vi "Autonomous Independent.vi"() -> ()   [LabVIEW 2015]
doc: "This VI is called when autonomous begins, and will automatically be terminated when autonomous ends. You can carry out timed or sensor driven robot movement independently without needing to return to the caller."
uses:
  <vilib>/Rock Robotics/WPI/Utilities/WPI_GetSetVariantRefNum.vi
  <vilib>/Rock Robotics/Network Tables/NT Write Numeric Array.vi
  <vilib>/Rock Robotics/Network Tables/NT Read String.vi
  <vilib>/Rock Robotics/WPI/RobotDrive/WPI_RobotDriveArcadeDrive_Standard(NoSaturation).vi
panel:
  out "Current Movement, for debugging":T1 {"Y Joystick Value" scale=1.0..-1.0; "X Joystick Value" scale=-1.0..1.0}
  in  "Array of robot movements":T2(array[cluster])=[{"X Joystick Value"=0.39393939393939403, "Y Joystick Value"=0.0, "Delay (sec)"=1.0, "Movement Name"="turn"}, {"X Joystick Value"=-0.3737373737373737, "Y Joystick Value"=0.0, "Delay (sec)"=1.0, "Movement Name"="turn back"}] {"Y Joystick Value" scale=1.0..-1.0; "X Joystick Value" scale=-1.0..1.0}
  # "Be sure to right-click and choose Data Operations>>Make Current Value default if you want to save the array values with the VI"
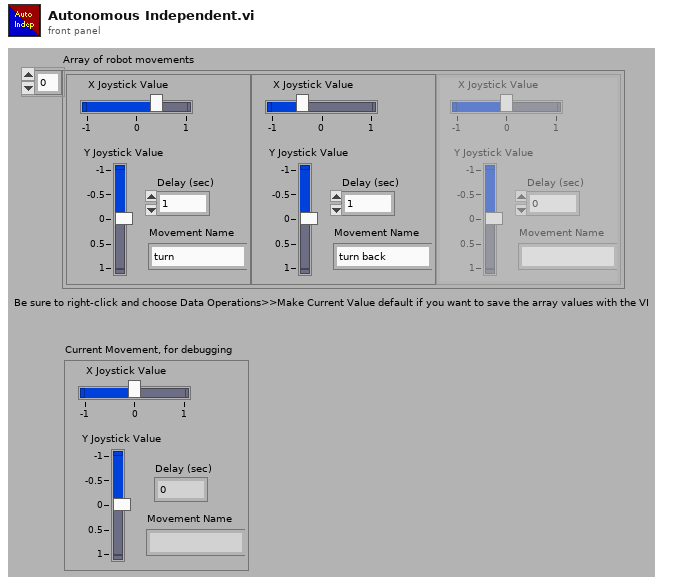
[diagram p1: front panel]
types:
  T1 = cluster{"X Joystick Value":dbl, "Y Joystick Value":dbl, "Delay (sec)":dbl, "Movement Name":string}
  T2 = cluster{"X Joystick Value":dbl, "Y Joystick Value":dbl, "Delay (sec)":dbl, "Movement Name":string}[]
  T3 = typedef "WPI_JoystickDevRef.ctl" = cluster{"Device":T4}
  T4 = typedef "WPI_JoystickDeviceEnum.ctl" = enum16{"USB 0", "USB 1", "USB 2", "USB 3", "USB 4", "USB 5"}
  T5 = typedef "WPI_RobotDriveDevRef.ctl" = cluster{"DevStatus":errorcluster, "Motors[]":T6[], "Square Inputs":bool, "Max Output":dbl}
  T6 = typedef "WPI_MotorControlDeviceRef.ctl" = cluster{"DeviceStatus":errorcluster, "Type":T7, "PWM":cluster{"PWM Channel":T8, "DeadBand":T9}, "CAN":cluster{"Device Number":u8, "Control Mode":T10, "Semaphore":T11, "Max Vout":dbl, "TalonSRX Control Mode":T12}, "Invert":bool}
  T7 = typedef "WPI_MotorControlType.ctl" = enum16{"PWM", "CAN", "CANTalonSRX"}
  T8 = typedef "FPGA_DIOPWMChannel.ctl" = enum8{"PWM 0", "PWM 1", "PWM 2", "PWM 3", "PWM 4", "PWM 5", "PWM 6", "PWM 7", "PWM 8", "PWM 9", "PWM MXP 0", "PWM MXP 1", "PWM MXP 2", "PWM MXP 3", "PWM MXP 4", "PWM MXP 5", "PWM MXP 6", "PWM MXP 7", "PWM MXP 8", "PWM MXP 9", "Invalid"}
  T9 = typedef "WPI_PWMDeadband.ctl" = cluster{"Name":string, "maxPositivePwm":i32, "minPositivePwm":i32, "centerPwm":i32, "maxNegativePwm":i32, "minNegativePwm":i32, "angularRange":u16}
  T10 = typedef "WPI_CANJaguar_ControlMode.ctl" = enum8{"Percent VBus", "Current", "Speed", "Position", "Voltage"}
  T11 = typedef "Semaphore RefNum" = refnum<k1>
  T12 = typedef "WPI_CANTalonSRX_APIControlMode.ctl" = enum8{"Percent VBus", "Speed", "Position", "Slave", "Unchanged / Invalid", "Voltage Compensation", "Current", "Motion Profile"}
  T13 = typedef "WPI_PotentiometerDevRef.ctl" = cluster{"DevStatus":errorcluster, "Analog Channel":T14, "Invert Output":bool}
  T14 = typedef "FPGA_AIChannel.ctl" = enum8{"AI 0", "AI 1", "AI 2", "AI 3", "AI MXP 0", "AI MXP 1", "AI MXP 2", "AI MXP 3", "Invalid"}
  T15 = typedef "WPI_SwitchDevRef.ctl" = cluster{"DevStatus":errorcluster, "DIO Channel":T16, "CntIndex":T17, "Normally Closed":bool}
  T16 = typedef "FPGA_DIOChannel.ctl" = enum8{"DIO 0", "DIO 1", "DIO 2", "DIO 3", "DIO 4", "DIO 5", "DIO 6", "DIO 7", "DIO 8", "DIO 9", "DIO MXP 0", "DIO MXP 1", "DIO MXP 2", "DIO MXP 3", "DIO MXP 4", "DIO MXP 5", "DIO MXP 6", "DIO MXP 7", "DIO MXP 8", "DIO MXP 9", "DIO MXP 10", "DIO MXP 11", "DIO MXP 12", "DIO MXP 13", "DIO MXP 14", "DIO MXP 15", "Invalid"}
  T17 = typedef "FPGA_CounterCtrSystemIndex.ctl" = enum8{"Ctr 0", "Ctr 1", "Ctr 2", "Ctr 3", "Ctr 4", "Ctr 5", "Ctr 6", "Ctr 7", "Invalid"}
  T18 = typedef "WPI_SolenoidDevRef.ctl" = cluster{"DevStatus":errorcluster, "Pneumatics Control Module":u8, "Forward Solenoid Channel":T19, "Reverse Solenoid Channel":T19}
  T19 = typedef "WPI_SolenoidChannel.ctl" = enum8{"Solenoid 0", "Solenoid 1", "Solenoid 2", "Solenoid 3", "Solenoid 4", "Solenoid 5", "Solenoid 6", "Solenoid 7", "Invalid"}
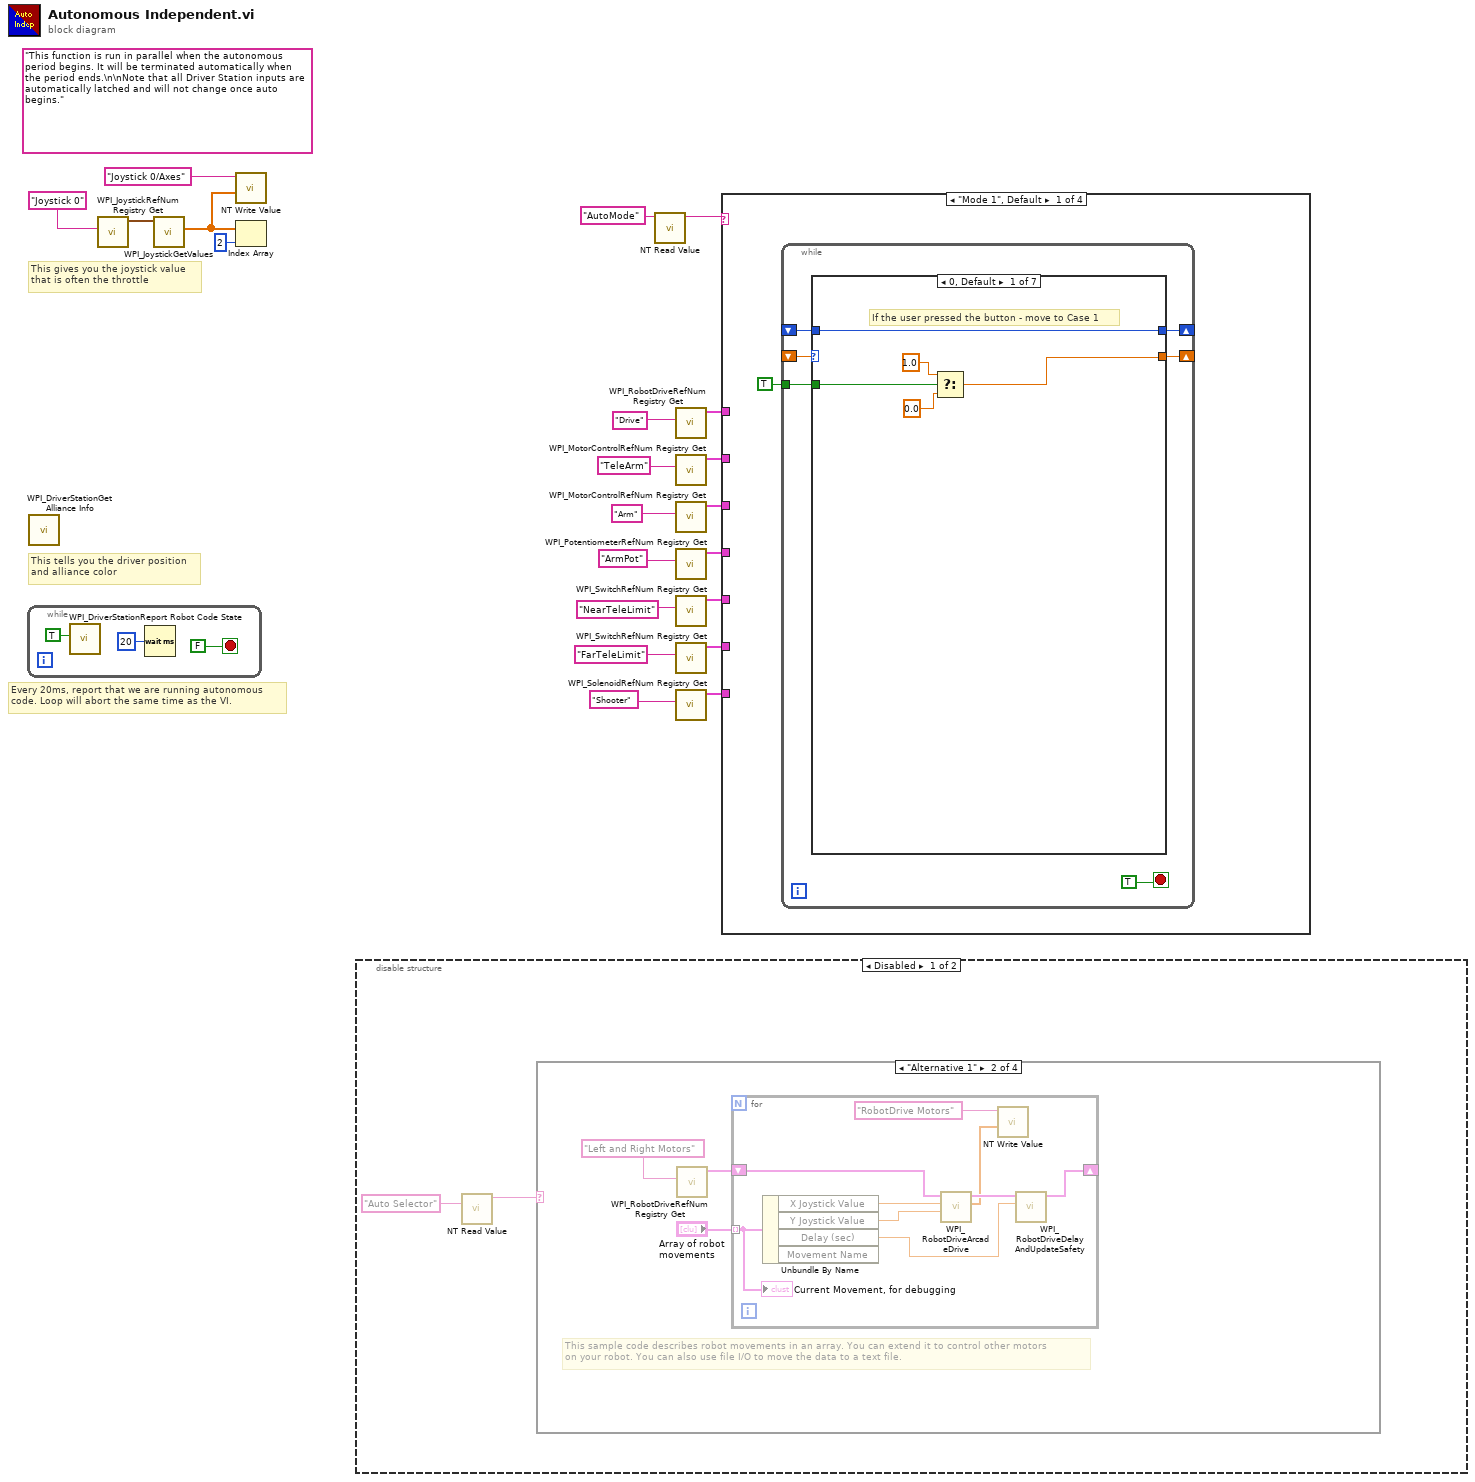
[diagram p0: block diagram]
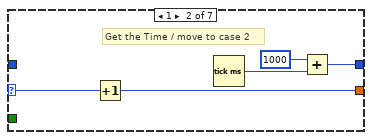
[diagram p2: hidden frame]
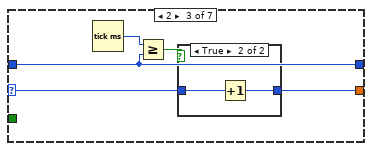
[diagram p3: hidden frame]
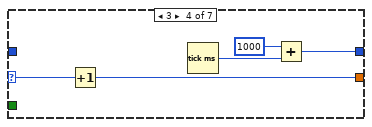
[diagram p5: hidden frame]
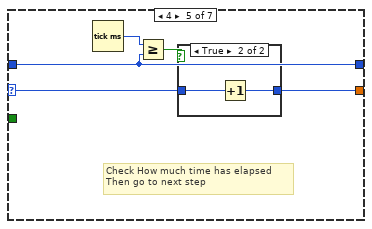
[diagram p6: hidden frame]
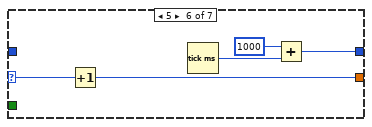
[diagram p8: hidden frame]
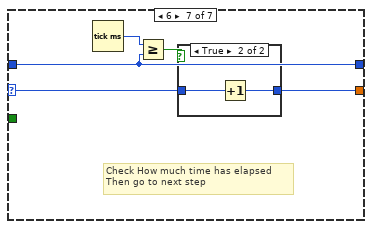
[diagram p9: hidden frame]
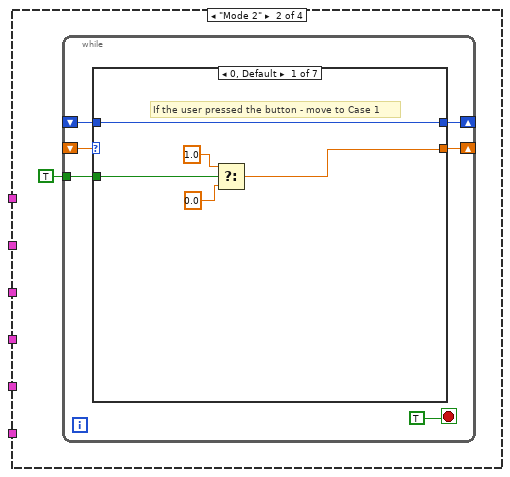
[diagram p11: hidden frame]
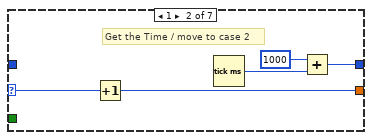
[diagram p12: hidden frame]
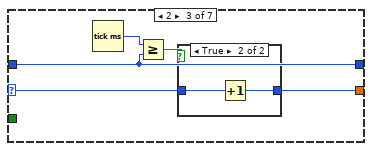
[diagram p13: hidden frame]
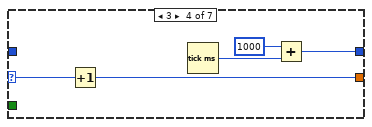
[diagram p15: hidden frame]
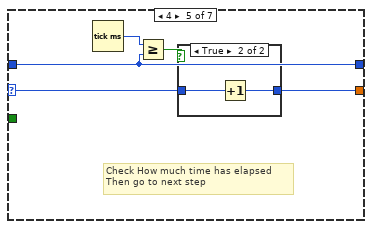
[diagram p16: hidden frame]
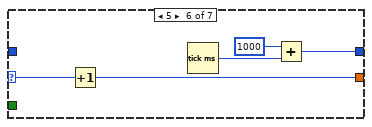
[diagram p18: hidden frame]
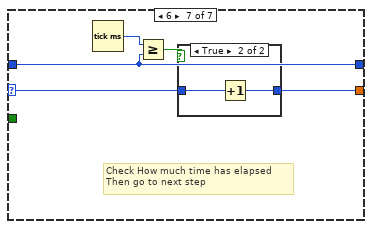
[diagram p19: hidden frame]
diagram:
  (unwired) "This function is run in parallel when the autonomous period begins. It will be terminated automatically when the period ends.\n\nNote that all Driver Station inputs are automatically latched and will not change once auto begins."
  # "Every 20ms, report that we are running autonomous\ncode. Loop will abort the same time as the VI."
  # "This gives you the joystick value\nthat is often the throttle"
  # "This tells you the driver position\nand alliance color"
  n1 = while {
    stop <- FALSE stop-if-true
    n2 = call <vilib>:"WPI_DriverStationReport Robot Code State.vi"("Autonomous"=TRUE) -> ()  [unwired: 10 in, 1 out]
    n3 = Wait (ms)(milliseconds to wait=u32 20) -> ()  [unwired: 1 out]
  }
  n4 = call <vilib>:"WPI_DriverStationGet Alliance Info.vi"() -> ()  [unwired: 12 out]
  n5 = call <vilib>:"WPI_JoystickRefNum Registry Get.vi"("refnum name"="Joystick 0") -> ("JoystickDevRef"=w20:T3)  [unwired: 1 in, 9 out]
  n6 = call <vilib>:"WPI_JoystickGetValues.vi"("JoystickDevRef"=w20) -> ("Axes"=w18:dbl[])  [unwired: 6 in, 4 out]
  n7 = call-poly <vilib>:"NT Write Value.vi"("Numeric Array"=w18, "Name"="Joystick 0/Axes") -> ()  [unwired: 9 in, 1 out]
  n8 = Index Array(array=w18, index=2) -> ()  [unwired: 1 out]
  n9 = disable-structure shown="Disabled" {
    frame Disabled {
      n10 = call-poly <vilib>:"NT Read Value.vi"("Name"="Auto Selector") -> ("String"=w25:string)  [unwired: 9 in, 1 out]
      n11 = case shown="\"Alternative 1\"" w25 {
        frame Default {
          # "You can put your main auto here, or you can right-click on the case and make any\nother frame be the default case."
          # "This is the frame that will execute if no selection is made, or if it is not recognized"
        }
        frame "Alternative 1" {
          # "This sample code describes robot movements in an array. You can extend it to control other motors\non your robot. You can also use file I/O to move the data to a text file."
          n12 = call <vilib>:"WPI_RobotDriveRefNum Registry Get.vi"("refnum name"="Left and Right Motors") -> ("RobotDriveDevRef"=w28:T5)  [unwired: 1 in, 9 out]
          n13 = for {
            shift-right: [w36] -> _
            shift-left: w28 -> [w37]
            tunnel: "Array of robot movements" -> [w32] mode=indexing
            n14 = Unbundle By Name(w32) -> ("X Joystick Value"=w35:dbl, "Y Joystick Value"=w34:dbl, "Delay (sec)"=w33:dbl)  [unwired: 1 out]
            n15 = call-poly <vilib>:"WPI_RobotDriveArcadeDrive.vi"("Y axis value"=w34, "X axis value"=w35, "RobotDriveDevRef"=w37) -> ("Motor Values"=w30:dbl[], "RobotDriveDevRef"=w38:T5)  [unwired: 1 in, 6 out]
            n16 = call-poly <vilib>:"NT Write Value.vi"("Numeric Array"=w30, "Name"="RobotDrive Motors") -> ()  [unwired: 9 in, 1 out]
            n17 = call <vilib>:"WPI_RobotDriveDelayAndUpdateSafety.vi"("Delay (s)"=w33, "RobotDriveDevRef"=w38) -> ("RobotDriveDevRef 2"=w36:T5)  [unwired: 8 in, 1 out]
            "Current Movement, for debugging" <- w32
          }
        }
        frame "Alternative 2" {
          w40 = "RobotDrive Motors" ("Name")
          # "This is some simple sample code to drive your robot curving one direction and then the other."
          # "stand still"
          # "other way for 0.5 second"
          # "turn for 1 second"
          n18 = call <vilib>:"WPI_RobotDriveRefNum Registry Get.vi"("refnum name"="Left and Right Motors") -> ("RobotDriveDevRef"=w56:T5)  [unwired: 1 in, 9 out]
          n19 = call-poly <vilib>:"WPI_RobotDriveArcadeDrive.vi"("Y axis value"=0.5 ("X axis value"), "X axis value"=-0.25, "RobotDriveDevRef"=w56) -> ("Motor Values"=w39:dbl[], "RobotDriveDevRef"=w49:T5)  [unwired: 1 in, 6 out]
          n20 = call-poly <vilib>:"NT Write Value.vi"("Numeric Array"=w39, "Name"=w40) -> ()  [unwired: 9 in, 1 out]
          n21 = call <vilib>:"WPI_RobotDriveDelayAndUpdateSafety.vi"("Delay (s)"=1.0, "RobotDriveDevRef"=w49) -> ("RobotDriveDevRef 2"=w50:T5)  [unwired: 8 in, 1 out]
          n22 = call-poly <vilib>:"WPI_RobotDriveArcadeDrive.vi"("Y axis value"=-0.25 ("X axis value"), "X axis value"=0.5, "RobotDriveDevRef"=w50) -> ("Motor Values"=w41:dbl[], "RobotDriveDevRef"=w51:T5)  [unwired: 1 in, 6 out]
          n23 = call-poly <vilib>:"NT Write Value.vi"("Numeric Array"=w41, "Name"=w40) -> ()  [unwired: 9 in, 1 out]
          n24 = call <vilib>:"WPI_RobotDriveDelayAndUpdateSafety.vi"("Delay (s)"=0.5, "RobotDriveDevRef"=w51) -> ("RobotDriveDevRef 2"=w52:T5)  [unwired: 8 in, 1 out]
          n25 = call-poly <vilib>:"WPI_RobotDriveArcadeDrive.vi"("Y axis value"=0.0 ("X axis value"), "X axis value"=0.0, "RobotDriveDevRef"=w52) -> ("Motor Values"=w42:dbl[])  [unwired: 1 in, 7 out]
          n26 = call-poly <vilib>:"NT Write Value.vi"("Numeric Array"=w42, "Name"=w40) -> ()  [unwired: 9 in, 1 out]
        }
        frame "Your Turn" {
        }
      }
    }
    frame Enabled {
    }
  }
  n27 = call-poly <vilib>:"NT Read Value.vi"("Name"="AutoMode") -> ("String"=w15:string)  [unwired: 9 in, 1 out]
  n28 = call <vilib>:"WPI_RobotDriveRefNum Registry Get.vi"("refnum name"="Drive") -> ("RobotDriveDevRef"=w7:T5)  [unwired: 9 in, 1 out]
  n29 = call <vilib>:"WPI_MotorControlRefNum Registry Get.vi"("refnum name"="TeleArm") -> ("MotorControlDevRef"=w6:T6)  [unwired: 9 in, 1 out]
  n30 = call <vilib>:"WPI_MotorControlRefNum Registry Get.vi"("refnum name"="Arm") -> ("MotorControlDevRef"=w5:T6)  [unwired: 9 in, 1 out]
  n31 = call <vilib>:"WPI_PotentiometerRefNum Registry Get.vi"("refnum name"="ArmPot") -> ("PotDevRef"=w4:T13)  [unwired: 9 in, 1 out]
  n32 = call <vilib>:"WPI_SwitchRefNum Registry Get.vi"("refnum name"="NearTeleLimit") -> ("SwitchDevRef"=w3:T15)  [unwired: 9 in, 1 out]
  n33 = call <vilib>:"WPI_SwitchRefNum Registry Get.vi"("refnum name"="FarTeleLimit") -> ("SwitchDevRef"=w2:T15)  [unwired: 9 in, 1 out]
  n34 = call <vilib>:"WPI_SolenoidRefNum Registry Get.vi"("refnum name"="Shooter") -> ("SolenoidDevRef"=w1:T18)  [unwired: 9 in, 1 out]
  n35 = case shown="\"Mode 1\", Default" w15 {
    tunnel: w7 -> [_ _ _ _]
    tunnel: w6 -> [_ _ _ _]
    tunnel: w5 -> [_ _ _ _]
    tunnel: w4 -> [_ _ _ _]
    tunnel: w3 -> [_ _ _ _]
    tunnel: w2 -> [_ _ _ _]
    tunnel: w1 -> [_ _ _ _]
    frame "Mode 1", Default {
      n36 = while {
        shift-right: [w62] -> _
        shift-left: _ -> [w61]
        shift-right: [w60] -> _
        shift-left: _ -> [w59]
        tunnel: TRUE -> [w58]
        stop <- TRUE stop-if-true
        n37 = case shown="0, Default" w61 {
          selector: w61 -> [_ w73 w77 w85 w90 w98 w103]
          tunnel: [w66 w72 w76 w84 w89 w97 w102] -> w62
          tunnel: [w65 w71 w74 w83 w87 w96 w100] -> w60
          tunnel: w59 -> [w65 _ w74 _ w87 _ w100]
          tunnel: w58 -> [w64 _ _ _ _ _ _]
          frame 0, Default {
            # "If the user pressed the button - move to Case 1"
            n38 = Select(t=1.0, s=w64, f=0.0) -> (s? t:f=w66:dbl)
          }
          frame 1 {
            # "Get the Time / move to case 2"
            n39 = Increment(x=w73) -> (x+1=w72:i32)
            n40 = Tick Count (ms)() -> (millisecond timer value=w70:u32)
            n41 = Add(x=u32 1000, y=w70) -> (x+y=w71:u32)
          }
          frame 2 {
            n42 = Tick Count (ms)() -> (millisecond timer value=w75:u32)
            n43 = Greater Or Equal?(x=w75, y=w74) -> (x >= y?=w78:bool)
            n44 = case shown="True" w78 {
              tunnel: [w79 w80] -> w76
              tunnel: w77 -> [w79 w81]
              frame False {
              }
              frame True {
                n45 = Increment(x=w81) -> (x+1=w80:i32)
              }
            }
          }
          frame 3 {
            n46 = Increment(x=w85) -> (x+1=w84:i32)
            n47 = Tick Count (ms)() -> (millisecond timer value=w86:u32)
            n48 = Add(x=u32 1000, y=w86) -> (x+y=w83:u32)
          }
          frame 4 {
            # "Check How much time has elapsed\nThen go to next step"
            n49 = Tick Count (ms)() -> (millisecond timer value=w88:u32)
            n50 = Greater Or Equal?(x=w88, y=w87) -> (x >= y?=w91:bool)
            n51 = case shown="True" w91 {
              tunnel: [w92 w93] -> w89
              tunnel: w90 -> [w92 w94]
              frame False {
              }
              frame True {
                n52 = Increment(x=w94) -> (x+1=w93:i32)
              }
            }
          }
          frame 5 {
            n53 = Increment(x=w98) -> (x+1=w97:i32)
            n54 = Tick Count (ms)() -> (millisecond timer value=w99:u32)
            n55 = Add(x=u32 1000, y=w99) -> (x+y=w96:u32)
          }
          frame 6 {
            # "Check How much time has elapsed\nThen go to next step"
            n56 = Tick Count (ms)() -> (millisecond timer value=w101:u32)
            n57 = Greater Or Equal?(x=w101, y=w100) -> (x >= y?=w104:bool)
            n58 = case shown="True" w104 {
              tunnel: [w105 w106] -> w102
              tunnel: w103 -> [w105 w107]
              frame False {
              }
              frame True {
                n59 = Increment(x=w107) -> (x+1=w106:i32)
              }
            }
          }
        }
      }
    }
    frame "Mode 2" {
      n60 = while {
        shift-right: [w113] -> _
        shift-left: _ -> [w112]
        shift-right: [w111] -> _
        shift-left: _ -> [w110]
        tunnel: TRUE -> [w109]
        stop <- TRUE stop-if-true
        n61 = case shown="0, Default" w112 {
          selector: w112 -> [_ w124 w128 w136 w141 w149 w154]
          tunnel: [w117 w123 w127 w135 w140 w148 w153] -> w113
          tunnel: [w116 w122 w125 w134 w138 w147 w151] -> w111
          tunnel: w110 -> [w116 _ w125 _ w138 _ w151]
          tunnel: w109 -> [w115 _ _ _ _ _ _]
          frame 0, Default {
            # "If the user pressed the button - move to Case 1"
            n62 = Select(t=1.0, s=w115, f=0.0) -> (s? t:f=w117:dbl)
          }
          frame 1 {
            # "Get the Time / move to case 2"
            n63 = Increment(x=w124) -> (x+1=w123:i32)
            n64 = Tick Count (ms)() -> (millisecond timer value=w121:u32)
            n65 = Add(x=u32 1000, y=w121) -> (x+y=w122:u32)
          }
          frame 2 {
            n66 = Tick Count (ms)() -> (millisecond timer value=w126:u32)
            n67 = Greater Or Equal?(x=w126, y=w125) -> (x >= y?=w129:bool)
            n68 = case shown="True" w129 {
              tunnel: [w130 w131] -> w127
              tunnel: w128 -> [w130 w132]
              frame False {
              }
              frame True {
                n69 = Increment(x=w132) -> (x+1=w131:i32)
              }
            }
          }
          frame 3 {
            n70 = Increment(x=w136) -> (x+1=w135:i32)
            n71 = Tick Count (ms)() -> (millisecond timer value=w137:u32)
            n72 = Add(x=u32 1000, y=w137) -> (x+y=w134:u32)
          }
          frame 4 {
            # "Check How much time has elapsed\nThen go to next step"
            n73 = Tick Count (ms)() -> (millisecond timer value=w139:u32)
            n74 = Greater Or Equal?(x=w139, y=w138) -> (x >= y?=w142:bool)
            n75 = case shown="True" w142 {
              tunnel: [w143 w144] -> w140
              tunnel: w141 -> [w143 w145]
              frame False {
              }
              frame True {
                n76 = Increment(x=w145) -> (x+1=w144:i32)
              }
            }
          }
          frame 5 {
            n77 = Increment(x=w149) -> (x+1=w148:i32)
            n78 = Tick Count (ms)() -> (millisecond timer value=w150:u32)
            n79 = Add(x=u32 1000, y=w150) -> (x+y=w147:u32)
          }
          frame 6 {
            # "Check How much time has elapsed\nThen go to next step"
            n80 = Tick Count (ms)() -> (millisecond timer value=w152:u32)
            n81 = Greater Or Equal?(x=w152, y=w151) -> (x >= y?=w155:bool)
            n82 = case shown="True" w155 {
              tunnel: [w156 w157] -> w153
              tunnel: w154 -> [w156 w158]
              frame False {
              }
              frame True {
                n83 = Increment(x=w158) -> (x+1=w157:i32)
              }
            }
          }
        }
      }
    }
    frame "Mode 3" {
      n84 = while {
        shift-right: [w164] -> _
        shift-left: _ -> [w163]
        shift-right: [w162] -> _
        shift-left: _ -> [w161]
        tunnel: TRUE -> [w160]
        stop <- TRUE stop-if-true
        n85 = case shown="0, Default" w163 {
          selector: w163 -> [_ w175 w179 w187 w192 w200 w205]
          tunnel: [w168 w174 w178 w186 w191 w199 w204] -> w164
          tunnel: [w167 w173 w176 w185 w189 w198 w202] -> w162
          tunnel: w161 -> [w167 _ w176 _ w189 _ w202]
          tunnel: w160 -> [w166 _ _ _ _ _ _]
          frame 0, Default {
            # "If the user pressed the button - move to Case 1"
            n86 = Select(t=1.0, s=w166, f=0.0) -> (s? t:f=w168:dbl)
          }
          frame 1 {
            # "Get the Time / move to case 2"
            n87 = Increment(x=w175) -> (x+1=w174:i32)
            n88 = Tick Count (ms)() -> (millisecond timer value=w172:u32)
            n89 = Add(x=u32 1000, y=w172) -> (x+y=w173:u32)
          }
          frame 2 {
            n90 = Tick Count (ms)() -> (millisecond timer value=w177:u32)
            n91 = Greater Or Equal?(x=w177, y=w176) -> (x >= y?=w180:bool)
            n92 = case shown="True" w180 {
              tunnel: [w181 w182] -> w178
              tunnel: w179 -> [w181 w183]
              frame False {
              }
              frame True {
                n93 = Increment(x=w183) -> (x+1=w182:i32)
              }
            }
          }
          frame 3 {
            n94 = Increment(x=w187) -> (x+1=w186:i32)
            n95 = Tick Count (ms)() -> (millisecond timer value=w188:u32)
            n96 = Add(x=u32 1000, y=w188) -> (x+y=w185:u32)
          }
          frame 4 {
            # "Check How much time has elapsed\nThen go to next step"
            n97 = Tick Count (ms)() -> (millisecond timer value=w190:u32)
            n98 = Greater Or Equal?(x=w190, y=w189) -> (x >= y?=w193:bool)
            n99 = case shown="True" w193 {
              tunnel: [w194 w195] -> w191
              tunnel: w192 -> [w194 w196]
              frame False {
              }
              frame True {
                n100 = Increment(x=w196) -> (x+1=w195:i32)
              }
            }
          }
          frame 5 {
            n101 = Increment(x=w200) -> (x+1=w199:i32)
            n102 = Tick Count (ms)() -> (millisecond timer value=w201:u32)
            n103 = Add(x=u32 1000, y=w201) -> (x+y=w198:u32)
          }
          frame 6 {
            # "Check How much time has elapsed\nThen go to next step"
            n104 = Tick Count (ms)() -> (millisecond timer value=w203:u32)
            n105 = Greater Or Equal?(x=w203, y=w202) -> (x >= y?=w206:bool)
            n106 = case shown="True" w206 {
              tunnel: [w207 w208] -> w204
              tunnel: w205 -> [w207 w209]
              frame False {
              }
              frame True {
                n107 = Increment(x=w209) -> (x+1=w208:i32)
              }
            }
          }
        }
      }
    }
    frame "Mode 4" {
      n108 = while {
        shift-right: [w215] -> _
        shift-left: _ -> [w214]
        shift-right: [w213] -> _
        shift-left: _ -> [w212]
        tunnel: TRUE -> [w211]
        stop <- TRUE stop-if-true
        n109 = case shown="0, Default" w214 {
          selector: w214 -> [_ w226 w230 w238 w243 w251 w256]
          tunnel: [w219 w225 w229 w237 w242 w250 w255] -> w215
          tunnel: [w218 w224 w227 w236 w240 w249 w253] -> w213
          tunnel: w212 -> [w218 _ w227 _ w240 _ w253]
          tunnel: w211 -> [w217 _ _ _ _ _ _]
          frame 0, Default {
            # "If the user pressed the button - move to Case 1"
            n110 = Select(t=1.0, s=w217, f=0.0) -> (s? t:f=w219:dbl)
          }
          frame 1 {
            # "Get the Time / move to case 2"
            n111 = Increment(x=w226) -> (x+1=w225:i32)
            n112 = Tick Count (ms)() -> (millisecond timer value=w223:u32)
            n113 = Add(x=u32 1000, y=w223) -> (x+y=w224:u32)
          }
          frame 2 {
            n114 = Tick Count (ms)() -> (millisecond timer value=w228:u32)
            n115 = Greater Or Equal?(x=w228, y=w227) -> (x >= y?=w231:bool)
            n116 = case shown="True" w231 {
              tunnel: [w232 w233] -> w229
              tunnel: w230 -> [w232 w234]
              frame False {
              }
              frame True {
                n117 = Increment(x=w234) -> (x+1=w233:i32)
              }
            }
          }
          frame 3 {
            n118 = Increment(x=w238) -> (x+1=w237:i32)
            n119 = Tick Count (ms)() -> (millisecond timer value=w239:u32)
            n120 = Add(x=u32 1000, y=w239) -> (x+y=w236:u32)
          }
          frame 4 {
            # "Check How much time has elapsed\nThen go to next step"
            n121 = Tick Count (ms)() -> (millisecond timer value=w241:u32)
            n122 = Greater Or Equal?(x=w241, y=w240) -> (x >= y?=w244:bool)
            n123 = case shown="True" w244 {
              tunnel: [w245 w246] -> w242
              tunnel: w243 -> [w245 w247]
              frame False {
              }
              frame True {
                n124 = Increment(x=w247) -> (x+1=w246:i32)
              }
            }
          }
          frame 5 {
            n125 = Increment(x=w251) -> (x+1=w250:i32)
            n126 = Tick Count (ms)() -> (millisecond timer value=w252:u32)
            n127 = Add(x=u32 1000, y=w252) -> (x+y=w249:u32)
          }
          frame 6 {
            # "Check How much time has elapsed\nThen go to next step"
            n128 = Tick Count (ms)() -> (millisecond timer value=w254:u32)
            n129 = Greater Or Equal?(x=w254, y=w253) -> (x >= y?=w257:bool)
            n130 = case shown="True" w257 {
              tunnel: [w258 w259] -> w255
              tunnel: w256 -> [w258 w260]
              frame False {
              }
              frame True {
                n131 = Increment(x=w260) -> (x+1=w259:i32)
              }
            }
          }
        }
      }
    }
  }
